vi "get_nextCellIndex.vi"(5 "which manipulator":T1(ring), 7 "unpatched cell indices ref":refnum<vi>, 8 "error in":errorcluster, 9 "transform cluster":T2, 10 "positions cluster":T3, 11 "current cell locations (px)":dbl[][](array[numeric])) -> (0 "error out":errorcluster, 2 "out of cells to patch":bool, 3 "next manip cell":i32)   [LabVIEW 2015]
uses:
  pipette cleaning/pressure box/cleaning_soft/controls/actuator_type.ctl
  pipette cleaning/pressure box/cleaning_soft/controls/actuator_cluster.ctl
  machine_vision/coordinate model vis/transform_properties_actuators.ctl
  machine_vision/controls/transform_cluster_actuator.ctl
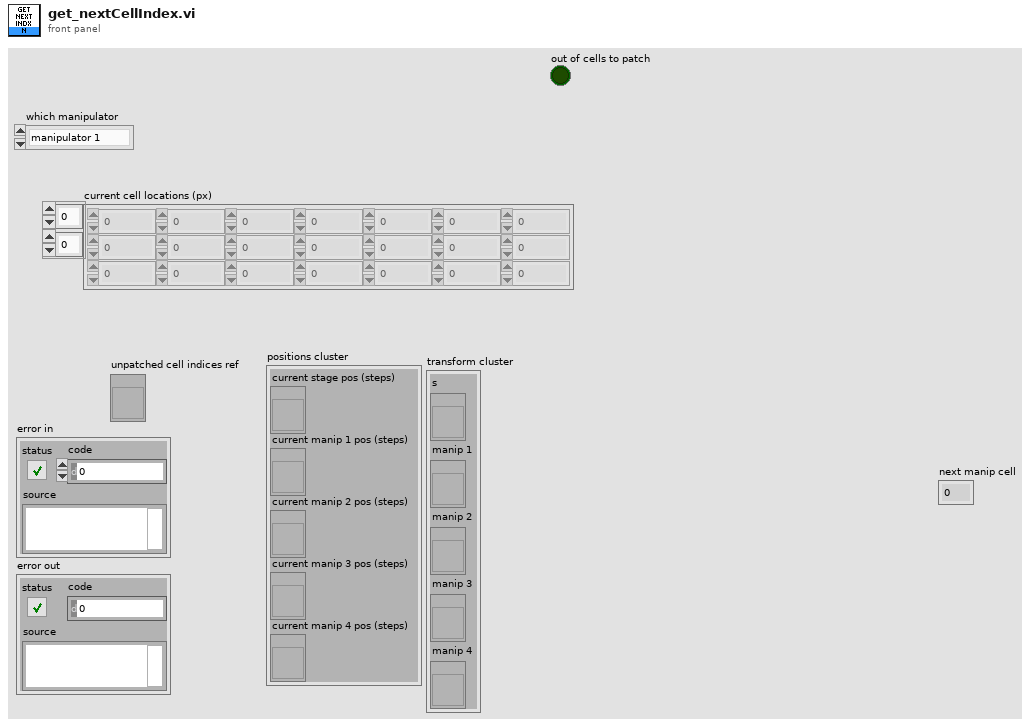
[diagram p1: front panel]
types:
  T1 = enum16{"manipulator 1", "manipulator 2", "manipulator 3", "manipulator 4"}
  T2 = typedef "transform_cluster_actuator.ctl" = cluster{"s":refnum<vi>, "manip 1":refnum<vi>, "manip 2":refnum<vi>, "manip 3":refnum<vi>, "manip 4":refnum<vi>}
  T3 = cluster{"current stage pos (steps)":refnum<vi>, "current manip 1 pos (steps)":refnum<vi>, "current manip 2 pos (steps)":refnum<vi>, "current manip 3 pos (steps)":refnum<vi>, "current manip 4 pos (steps)":refnum<vi>}
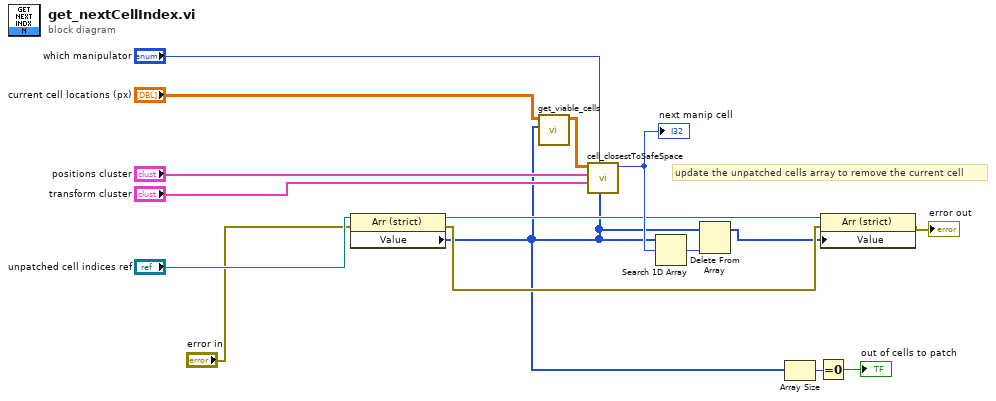
[diagram p0: block diagram]
diagram:
  # "update the unpatched cells array to remove the current cell"
  n1 = property on="Property Node" class="Arr (strict)"(reference="unpatched cell indices ref", error in="error in") -> (reference out=w10:refnum<vi>, error out=w6:errorcluster, "Value"=w1:i32[])
  n2 = call "get_viable_cells.vi"("cell indices"=w1, "current cell locations (px)"="current cell locations (px)") -> ("viable cell locations (px)"=w13:dbl[][])  [unwired: 9 in]
  n3 = call "cell_closestToSafeSpace.vi"("manip 1 cell indices"=w1, "which manipulator"="which manipulator", "transform cluster + actuator"="transform cluster", "current positions"="positions cluster", "current cell locations (px)"=w13) -> ("closest cell index"=w16:i32)  [unwired: 5 in, 1 out]
  "next manip cell" <- w16
  n4 = Search 1D Array(1D array=w1, element=w16) -> (index of element=w15:i32)  [unwired: 1 in]
  n5 = Delete From Array(array=w1, index=w15) -> (array with subset deleted=w2:i32[])  [unwired: 1 in, 1 out]
  n6 = Array Size(array=w1) -> (size(s)=w4:i32)
  n7 = Equal To 0?(x=w4) -> (x = 0?=→"out of cells to patch":bool)
  n8 = property on="Property Node" class="Arr (strict)"(reference=w10, error in=w6, "Value"=w2) -> (error out=→"error out":errorcluster)  [unwired: 1 out]
